vi "FRCts20_WebMethods_SingleEvent_GET.vi"(7 "httpRequestID":u32, 8 "Event":string, 9 "View":string) -> ()   [LabVIEW 2014, in "FRCts20_WebMethods.lvlib"]
uses:
  FRCts20_WebMethods.lvlib
  Backend/source/VI Source/FRCts20_Backend_API/FRCts20_Backend_API_Command_Event.ctl
  Backend/source/VI Source/FRCts20_Backend_API/FRCts20_Backend_API_Event.ctl
  Backend/source/VI Source/FRCts20_Backend_API/FRCts20_Backend_API_SW.ctl
  Backend/source/VI Source/FRCts20_Backend_API/FRCts20_Backend_API_Command_ClosedRequests.ctl
  Backend/source/VI Source/FRCts20_Backend_API/FRCts20_Backend_API_ClosedRequests.ctl
  Backend/source/VI Source/FRCts20_Backend_API/FRCts20_Backend_API_Event.vi
  Backend/source/VI Source/FRCts20_Backend_API/FRCts20_Backend_API_ClosedRequests.vi
  ESP Engine/source/VI Source/FRCts20_EspEngine.lvlib
  Backend/source/VI Source/FRCts20_Backend_API/FRCts20_Backend_API.lvlib
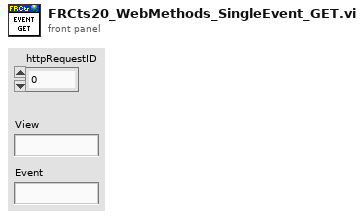
[diagram p1: front panel]
types:
  T1 = typedef "FRCts20_Backend_API.lvlib/FRCts20_Backend_API_ClosedRequests.ctl" = cluster{"Event Name":string, "APIReturn":string, "Array of Requests":cluster{"Team Number":string, "ReqNumber":string, "Request":string, "OpenDate":string, "CloseDate":string}[]}
  T2 = typedef "FRCts20_Backend_API.lvlib/FRCts20_Backend_API_Command_ClosedRequests.ctl" = string
  T3 = typedef "FRCts20_Backend_API.lvlib/FRCts20_Backend_API_Event.ctl" = cluster{"Event Index":u32, "Name":string, "Start Time":timestamp, "End Time":timestamp, "Teams":cluster{"Team Index":u32, "Team Number":u32, "Requests":cluster{"Request Number":u32, "Description":string}[], "Has Open Issue":bool}[], "SWType":T4, "APIReturn":string}
  T4 = typedef "FRCts20_Backend_API.lvlib/FRCts20_Backend_API_SW.ctl" = string
  T5 = typedef "FRCts20_Backend_API.lvlib/FRCts20_Backend_API_Command_Event.ctl" = string
  T6 = typedef "FRCts20_EspEngine.lvlib/FRCts20_EspEngine_SearchBrowser.ctl" = cluster{"Event":cluster{"Event Index":u32, "Event Name":string, "Start Time":timestamp, "End Time":timestamp, "OpenIssues":u8, "IsLive":bool}[], "select-choice-software":string, "select-choice-location":string}
  T7 = typedef "FRCts20_EspEngine.lvlib/FRCts20_EspEngine_Event.ctl" = cluster{"Single Event":T8, "EventOpenIssueCount":i16, "Requests":cluster{"RequestId":i32, "Request Description":string, "Team Number":i32}[], "ClosedRequests":cluster{"RequestId":i32, "Request Description":string, "Team Number":i32}[], "NotFoundStatus":bool}
  T8 = typedef "FRCts20_WebMethods.lvlib/FRCts20_WebMethods_ctl_singleEvent.ctl" = cluster{"Team":T9[], "Issue Count":i32, "Location":string, "Start Date ":timestamp}
  T9 = typedef "FRCts20_WebMethods.lvlib/FRCts20_WebMethods_ctl_teamIdentifier.ctl" = cluster{"Team Nickname":string, "Team Number ":u32, "UniqueId":u32}
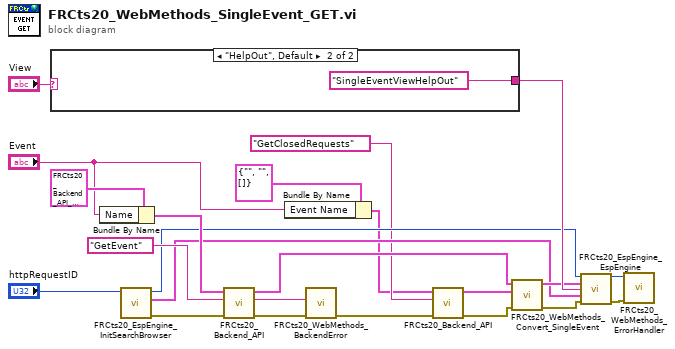
[diagram p0: block diagram]
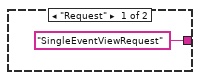
[diagram p2: hidden frame]
diagram:
  n1 = case shown="\"HelpOut\", Default" "View" {
    tunnel: ["SingleEventViewRequest" "SingleEventViewHelpOut"] -> w22
    frame "Request" {
    }
    frame "HelpOut", Default {
    }
  }
  n2 = Bundle By Name(cluster=T3 {"Event Index"=0, "Name"="", "Start Time"=timestamp(0 s since 1904-01-01), "End Time"=timestamp(0 s since 1904-01-01), "Teams"=[], "SWType"="", "APIReturn"=""} ("Event In"), "Name"="Event") -> (w19:T3)
  n3 = call "FRCts20_EspEngine_InitSearchBrowser.vi"("httpRequestID"="httpRequestID") -> ("error out"=w9:errorcluster, "SearchBrowser"=w8:T6, "httpRequestID out"=w10:u32)  [unwired: 8 in]
  n4 = call-poly "FRCts20_Backend_API.vi"("error in (no error)"=w9, "Command"=T5 "GetEvent", "Event In"=w19) -> ("error out"=w18:errorcluster, "Status"=w15:string, "Event Out"=w14:T3)  [unwired: 6 in]
  n5 = Bundle By Name(cluster=T1 {"Event Name"="", "APIReturn"="", "Array of Requests"=[]} ("DataIn"), "Event Name"="Event") -> (w1:T1)
  n6 = call "FRCts20_WebMethods_BackendError.vi"("error in (no error)"=w18, "Status"=w15) -> ("error out"=w6:errorcluster)  [unwired: 8 in, 1 out]
  n7 = call-poly "FRCts20_Backend_API.vi"("error in (no error)"=w6, "Command"=T2 "GetClosedRequests", "DataIn"=w1) -> ("error out"=w5:errorcluster, "DataOut"=w4:T1)  [unwired: 6 in, 1 out]
  n8 = call "FRCts20_WebMethods_Convert_SingleEvent.vi"("error in (no error)"=w5, "ClosedRequestsData"=w4, "Event Out"=w14) -> ("error out"=w12:errorcluster, "Event"=w13:T7)  [unwired: 7 in]
  n9 = call "FRCts20_EspEngine_EspEngine.vi"("httpRequestID"=w10, "Cluster"=w13, "Page"=w22, "SearchBrowser"=w8, "error in (no error)"=w12) -> ("httpRequestID out"=w16:u32, "error out"=w17:errorcluster)  [unwired: 9 in]
  n10 = call "FRCts20_WebMethods_ErrorHandler.vi"("error in"=w17, "httpRequestID"=w16) -> ()  [unwired: 9 in, 1 out]
